vi "LEDDebugColorSensors.vi"(5 "LED Length":i32=12, 7 "Value":dbl, 9 "Max":dbl, 11 "Min":dbl, 12 "Background Color":u32(colorbox)=16711680, 13 "Color to Insert":u32(colorbox)=16711680) -> (6 "Output Color Array":u32[](array[numeric]))   [LabVIEW 2019]
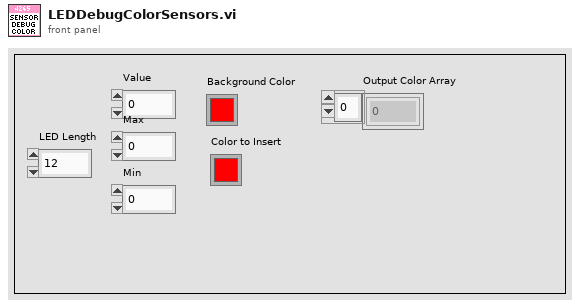
[diagram p1: front panel]
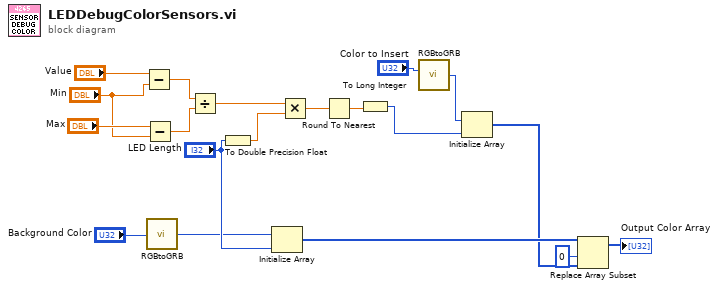
[diagram p0: block diagram]
diagram:
  n1 = Subtract(x="Value", y="Min") -> (x-y=w9:dbl)
  n2 = Subtract(x="Max", y="Min") -> (x-y=w8:dbl)
  n3 = call "RGBtoGRB.vi"("Color (RGB)"="Background Color") -> ("Color (GRB)"=w3:u32)
  n4 = Divide(x=w9, y=w8) -> (x/y=w19:dbl)
  n5 = To Double Precision Float(number="LED Length") -> (double precision float=w18:dbl)
  n6 = Initialize Array(w3, "LED Length") -> (w14:u32[])
  n7 = Multiply(x=w19, y=w18) -> (x*y=w17:dbl)
  n8 = Round To Nearest(number=w17) -> (nearest integer value=w16:dbl)
  n9 = To Long Integer(number=w16) -> (32bit integer=w7:i32)
  n10 = call "RGBtoGRB.vi"("Color (RGB)"="Color to Insert") -> ("Color (GRB)"=w5:u32)
  n11 = Initialize Array(w5, w7) -> (w1:u32[])
  n12 = Replace Array Subset(array=w14, new element=w1, index=0) -> (→"Output Color Array":u32[])
